vi "Pressure to Caller.vi"(8 "error in (no error)":errorcluster, 10 "Analog Input Waveform":waveform(dbl), 11 "Baratron in":refnum<class "Baratron.lvclass">) -> (0 "error out":errorcluster)   [LabVIEW 2021, in "Baratron.lvclass"]
uses:
  Baratron.lvclass
  C:/Program Files/National Instruments/LabVIEW 2021/vi.lib/ActorFramework/Actor/Actor.lvclass
  Baratron.lvclass/Baratron.ctl
  <vilib>/ActorFramework/Actor/Actor.lvclass/Actor.ctl
  Pressure Gauges/Pressure Gauges Messages/Received Pressure Msg/Received Pressure Msg.lvclass/Received Pressure Msg.ctl
  <vilib>/ActorFramework/Message Enqueuer/Message Enqueuer.lvclass/Message Enqueuer.ctl
  <vilib>/ActorFramework/Message Enqueuer/Enqueue.vi
  Pressure Gauges/Pressure Gauges Messages/Received Pressure Msg/Received Pressure Msg.lvclass
  C:/Program Files/National Instruments/LabVIEW 2021/vi.lib/ActorFramework/Message/Message.lvclass
  <vilib>/ActorFramework/Message Priority Queue/Priority Enqueue.vi
  <vilib>/ActorFramework/Actor/Actor.lvclass
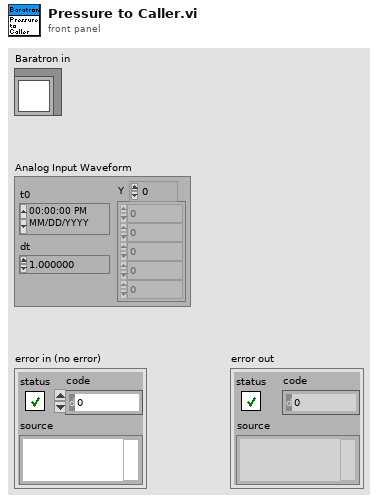
[diagram p1: front panel]
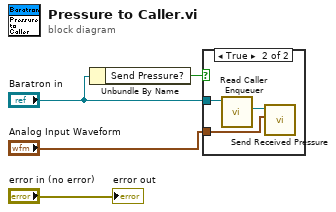
[diagram p0: block diagram]
diagram:
  n1 = Unbundle By Name("Baratron in") -> ("Send Pressure?"=w3:bool)
  n2 = case shown="True" w3 {
    tunnel: "Baratron in" -> [_ w7]
    tunnel: "Analog Input Waveform" -> [_ w5]
    frame False {
    }
    frame True {
      n3 = call <vilib>:"Read Caller Enqueuer.vi"("Actor"=w7) -> ("Caller Enqueuer"=w6:refnum<class "Message Enqueuer.lvclass">)  [unwired: 10 in]
      n4 = call "Send Received Pressure.vi"("Received Pressure"=w5, "Message Enqueuer"=w6) -> ()  [unwired: 8 in, 2 out]
    }
  }
  "error out" <- "error in (no error)"
